vi "FVer (Read).vi"(6 "ISOBUS address":T2=-1 caption="ISOBUS address (-1)", 8 "error in":errorcluster, 11 "Mercury Reference In":T3) -> (0 "error out":errorcluster, 2 "Firmware Version":string, 3 "Mercury Reference Out":T3, 4 "Valid?":T1)   [LabVIEW 2018, in "Mercury iXX.lvlib" / "Auxiliary.lvlib"]
doc: "Returns the firmware version of the selected device."
uses:
  Auxiliary.lvlib
  Mercury Reference.ctl
  Comms Transport Layer.ctl
  Query Dynamic Reference.ctl
  ISOBus Address.ctl
  Is Valid LED.ctl
  Command Verbs.ctl
  Mercury iXX.lvlib
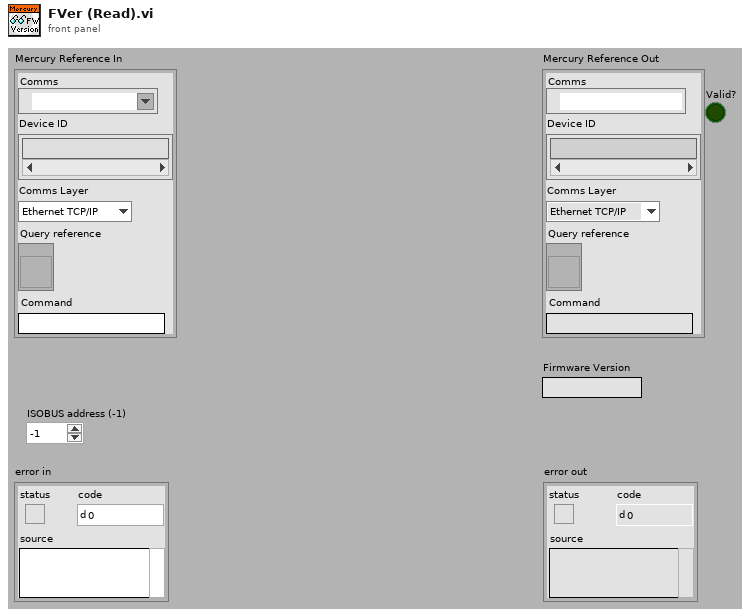
[diagram p1: front panel]
types:
  T1 = typedef "Mercury iXX.lvlib/Is Valid LED.ctl" = bool
  T2 = typedef "Mercury iXX.lvlib/ISOBus Address.ctl" = i32
  T3 = typedef "Mercury iXX.lvlib/Mercury Reference.ctl" = cluster{"Comms":refnum<visa-resource-name>, "Device ID":string[], "Comms Layer":T4, "Command":string, "Query reference":T5}
  T4 = typedef "Mercury iXX.lvlib/Comms Transport Layer.ctl" = enum16{"Ethernet TCP/IP", "USB", "ISOBus - RS-232", "GPIB"}
  T5 = typedef "Mercury iXX.lvlib/Query Dynamic Reference.ctl" = refnum<vi>
  T6 = typedef "Mercury iXX.lvlib/Command Verbs.ctl" = string
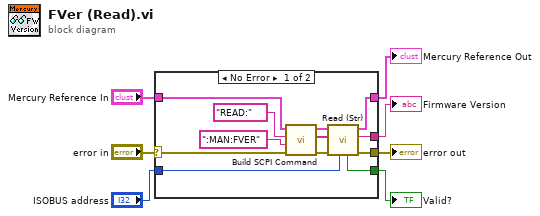
[diagram p0: block diagram]
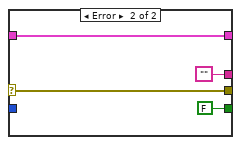
[diagram p2: hidden frame]
diagram:
  n1 = case shown="No Error" "error in" {
    selector: "error in" -> [w9 w22]
    tunnel: "Mercury Reference In" -> [w10 w23]
    tunnel: [w11 w23] -> w6
    tunnel: [w8 w22] -> w5
    tunnel: "ISOBUS address" -> [w14 _]
    tunnel: [w12 ""] -> w2
    tunnel: [w13 FALSE ("Valid?")] -> w1
    frame No Error {
      n2 = call "Build SCPI Command.vi"("error in"=w9, "Noun(s)"=":MAN:FVER" ("Command"), "Verb"=T6 "READ:", "Mercury Reference In"=w10) -> ("error out"=w15:errorcluster, "SCPI Message(s)"=w16:string[], "Mercury Reference Out"=w17:T3)  [unwired: 5 out]
      n3 = call "Read (Str).vi"("ISOBUS address"=w14, "error in"=w15, "SCPI Message(s)"=w16, "Mercury Reference In"=w17) -> ("error out"=w8:errorcluster, "Response"=w12:string, "Mercury Reference Out"=w11:T3, "Valid?"=w13:T1)  [unwired: 4 out]
    }
    frame Error {
    }
  }
  "Mercury Reference Out" <- w6
  "error out" <- w5
  "Firmware Version" <- w2
  "Valid?" <- w1
